vi "connect.vi"(8 "error in (no error)":errorcluster, 11 "SEDSpectrometer in":refnum<class "FiberSpectrograph.lvclass">) -> (0 "error out":errorcluster, 2 "Connected":bool, 3 "SEDSpectrometer out":refnum<class "FiberSpectrograph.lvclass">)   [LabVIEW 2016, in "FiberSpectrograph.lvclass"]
uses:
  FiberSpectrograph.lvclass
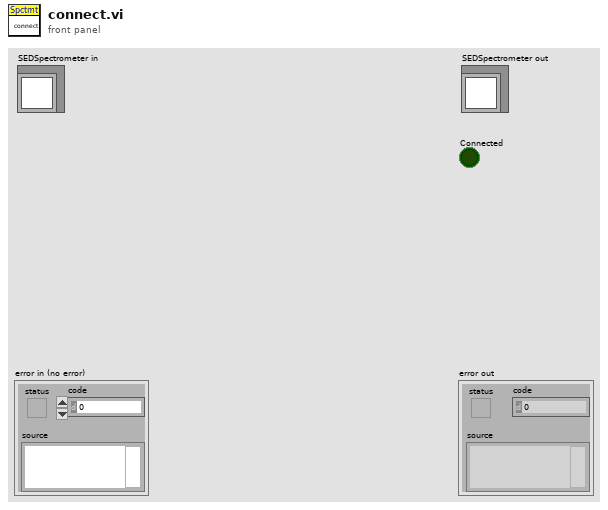
[diagram p1: front panel]
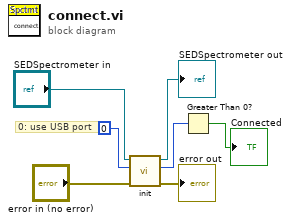
[diagram p0: block diagram]
diagram:
  # "0: use USB port"
  n1 = call "init.vi"("error in (no error)"="error in (no error)", "Port"=0, "SEDSpectrometer in"="SEDSpectrometer in") -> ("error out"=→"error out":errorcluster, "Output Value"=w6:i32, "SEDSpectrometer out"=→"SEDSpectrometer out":refnum<class "FiberSpectrograph.lvclass">)  [unwired: 6 in]
  n2 = Greater Than 0?(x=w6) -> (x > 0?=→"Connected":bool)
